vi "trash_Write Timestamps.vi"(8 "error in (no error)":errorcluster, 9 "Time":u64, 10 "Timestamp":T1, 11 "CIFTemplateNode in":refnum<class "CIFCorePlugin.lvclass">) -> (0 "error out":errorcluster, 3 "CIFTemplateNode out":refnum<class "CIFCorePlugin.lvclass">)   [LabVIEW 2021]
doc: "Update Timestamp for Plug-in statistics.\n\nA value of 0 for the Time input will cause the VI to get the current timestamp."
uses:
  CIFUtilities/CIFClocks/CIFClocks.lvlib
  CIFCorePlugin.lvclass
  CIFCoreCommon/Typedef/Plugin Timestamp Enum.ctl
  CIFCoreCommon/CIFCoreCommon.lvlib
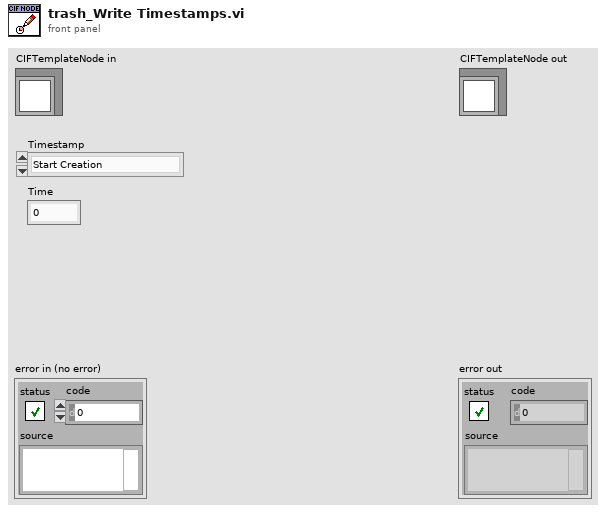
[diagram p1: front panel]
types:
  T1 = typedef "CIFCoreCommon.lvlib/Plugin Timestamp Enum.ctl" = enum32{"Start Creation", "Start gRPC Servers", "Start Listening", "Start Running", "Wake", "Start Execute", "Read FIFO", "Write Output", "Cycle Execute", "Start Housekeeping", "Start Sleep", "Start Cleaningup", "Start Destroying"}
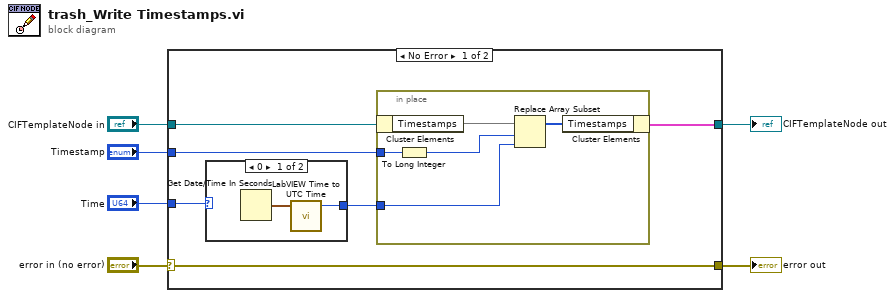
[diagram p0: block diagram]
diagram:
  n1 = case shown="No Error" "error in (no error)" {
    selector: "error in (no error)" -> [w12 w21]
    tunnel: [w12 w21] -> w5
    tunnel: [w9 w22] -> w3
    tunnel: "CIFTemplateNode in" -> [w10 w22]
    tunnel: "Time" -> [w11 _]
    tunnel: "Timestamp" -> [w7 _]
    frame No Error {
      n2 = case shown="0" w11 {
        selector: w11 -> [_ w20]
        tunnel: [w18 w20] -> w8
        frame 0 {
          n3 = Get Date/Time In Seconds() -> (seconds since 1Jan1904=w19:timestamp)
          n4 = call "LabVIEW Time to UTC Time.vi"("LabVIEW Time (s)"=w19) -> ("UTC Time (ns)"=w18:u64)  [unwired: 4 in]
        }
        frame 1, Default {
        }
      }
      n5 = in-place {
        in-place-border: w8 -> [w16]
        in-place-border: w7 -> [w15]
        n6 = in-place-cluster #1(w10) -> ("Timestamps"=w17)
        n7 = To Long Integer(number=w15) -> (32bit integer=w14:i32)
        n8 = Replace Array Subset(array=w17, new element=w16, index=w14) -> (w13:u64[])
        n9 = in-place-cluster #1("Timestamps"=w13) -> (w9:cluster{})
      }
    }
    frame Error {
    }
  }
  "error out" <- w5
  "CIFTemplateNode out" <- w3
